vi "test_data-type.vi"() -> ()   [LabVIEW 2019]
uses:
  <vilib>/Utility/miscctls.llb/LV3DPointTypeDef.ctl
  <vilib>/picture/3D Picture Control/Object/Create Object (drawable).vi
  <vilib>/picture/3D Picture Control/Object/Add Object (no reference).vi
  <vilib>/picture/3D Picture Control/Helpers/Set Light (no reference).vi
  <vilib>/picture/3D Picture Control/NI_3D Picture Control.lvlib
panel:
  in  "Color":u32(colorbox)=16711680
  in  "N of slice":u32=128
  in  "dt":u32=50
  in  "stop":bool
  out "3D Picture":refnum<vi>(3d-picture)
  in  "Draw Mode":T1(ring)
  in  "Size":dbl(slide) scale=0.0..10.0
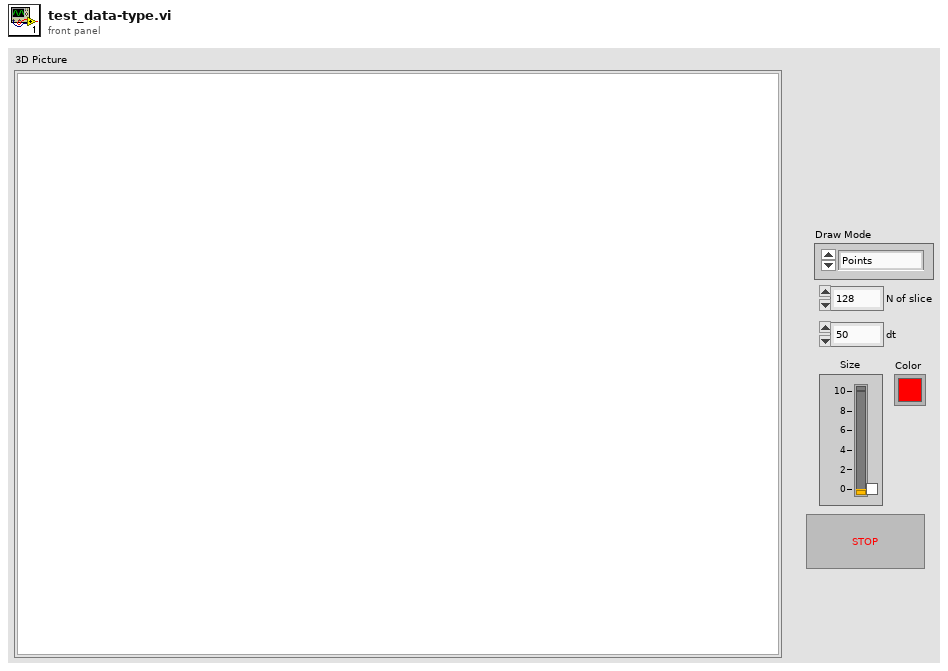
[diagram p1: front panel]
types:
  T1 = enum16{"Points", "Lines", "Line Strip", "Line Loop", "Triangles", "Triangle Strip", "Triangle Fan", "Quads", "Quad Strip", "Polygon"}
  T2 = enum16{"Inherit Value", "Points", "Wireframe", "Polygons"}
  T3 = typedef "LV3DPointTypeDef.ctl" = cluster{"X":sgl, "Y":sgl, "Z":sgl}
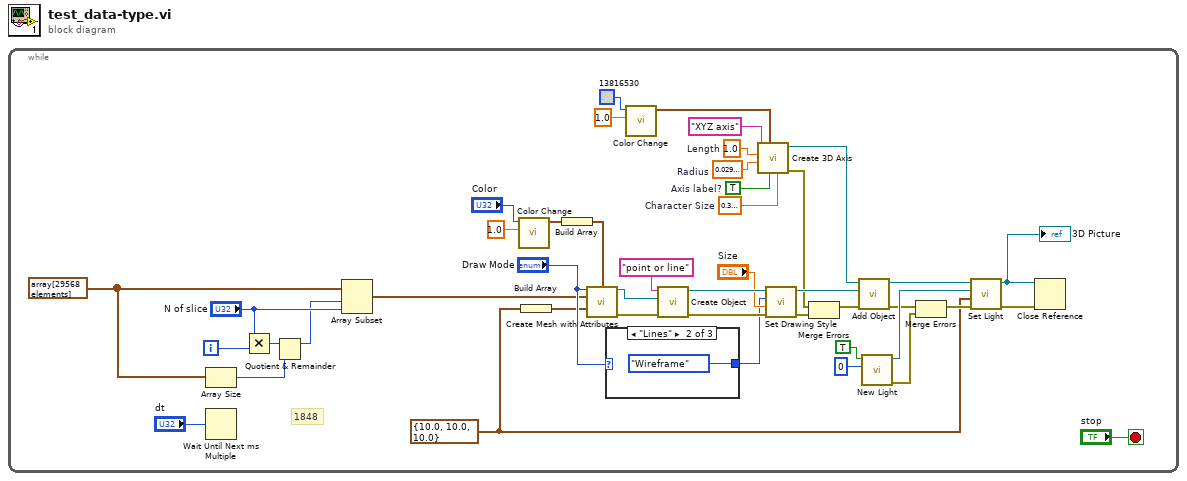
[diagram p0: block diagram]
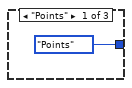
[diagram p2: hidden frame]
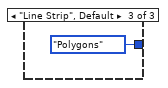
[diagram p3: hidden frame]
diagram:
  n1 = while {
    i -> [w6]
    stop <- "stop" stop-if-true
    w5 = cluster{"x":dbl, "y":dbl, "z":dbl}[] array[29568 elements] ("Array")
    w13 = sgl 0.3  # Character Size
    w12 = T3 {"X"=10.0, "Y"=10.0, "Z"=10.0} ("Position")
    w32 = sgl 1.0  # Length
    w36 = sgl 0.03  # Radius
    w37 = TRUE  # Axis label?
    # "1848"
    n2 = Array Size(array=w5) -> (size(s)=w2:i32)
    n3 = Wait Until Next ms Multiple(millisecond multiple="dt") -> ()  [unwired: 1 out]
    n4 = Multiply(x="N of slice", y=w6) -> (x*y=w3:u32)
    n5 = Quotient & Remainder(x=w3, y=w2) -> (x-y*floor(x/y)=w1:u32)  [unwired: 1 out]
    n6 = Array Subset(array=w5, index=w1, length="N of slice") -> (w7:cluster{"x":dbl, "y":dbl, "z":dbl}[])
    n7 = call <vilib>:"Color Change.vi"("Alpha"=1.0, "Color"="Color") -> ("RGBA"=w41:cluster{"R":sgl, "G":sgl, "B":sgl, "A":sgl})  [unwired: 9 in]
    n8 = Build Array(w12) -> (w11:T3[])
    n9 = Build Array(w41) -> (w40:cluster{"R":sgl, "G":sgl, "B":sgl, "A":sgl}[])
    n10 = call <vilib>:"Create Mesh with Attributes.vi"("Draw Mode"="Draw Mode", "Color Array"=w40, "Vertex Array"=w7, "Normal Array"=w11) -> ("New Mesh Refnum"=w44:refnum<vi>, "error out"=w43:errorcluster)  [unwired: 10 in]
    n11 = case shown="\"Lines\"" "Draw Mode" {
      tunnel: [T2."Points" ("Mode") T2."Wireframe" ("Mode") T2."Polygons" ("Mode")] -> w14
      frame "Points" {
      }
      frame "Lines" {
      }
      frame "Line Strip", Default {
      }
    }
    n12 = call <vilib>:"Color Change.vi"("Alpha"=1.0, "Color"=u32 13816530) -> ("RGBA"=w33:cluster{"R":sgl, "G":sgl, "B":sgl, "A":sgl})  [unwired: 9 in]
    n13 = call-poly <vilib>:"Create Object.vi"("error in (no error)"=w43, "Geometry"=w44, "Name"="point or line") -> ("error out"=w25:errorcluster, "Scene:New Object"=w27:refnum<vi>)  [unwired: 7 in]
    n14 = call <vilib>:"Create 3D Axis.vi"("Character Size"=w13, "Axis label?"=w37, "Color"=w33, "Radius"=w36, "Length"=w32, "Name"="XYZ axis") -> ("error out"=w19:errorcluster, "New Object Refnum"=w20:refnum<vi>)  [unwired: 4 in]
    n15 = call <vilib>:"Set Drawing Style.vi"("error in (no error)"=w25, "Size"="Size", "Mode"=w14, "Scene Object In"=w27) -> ("error out"=w24:errorcluster, "Scene Object Out"=w26:refnum<vi>)  [unwired: 6 in]
    n16 = Merge Errors(w19, w24) -> (w22:errorcluster)
    n17 = call-poly <vilib>:"Add Object.vi"("error in (no error)"=w22, "New Object In"=w26, "Scene Object In"=w20) -> ("error out"=w18:errorcluster, "Scene Object Out"=w31:refnum<vi>)  [unwired: 7 in]
    n18 = call <vilib>:"New Light.vi"("Light Number"=0, "At Infinity"=TRUE) -> ("error out"=w16:errorcluster, "New Light Refnum"=w30:refnum<vi>)  [unwired: 8 in]
    n19 = Merge Errors(w18, w16) -> (w17:errorcluster)
    n20 = call-poly <vilib>:"Set Light.vi"("error in (no error)"=w17, "Position"=w12, "Light Refnum In"=w30, "Scene Object In"=w31) -> ("error out"=w10:errorcluster, "Scene Object Out"=w9:refnum<vi>)  [unwired: 6 in]
    "3D Picture" <- w9
    n21 = Close Reference(reference=w9, error in (no error)=w10) -> ()  [unwired: 1 out]
  }
